vi "Mixed Mode Parameters Dialog.vi"(8 "error in (no error)":errorcluster, 11 "LBCB":T2) -> (0 "error out":errorcluster)   [LabVIEW 2009]
uses:
  lib/Data Access Objects/Metadata/Cartesian Point.ctl
  lib/Data Access Objects/Metadata/Cartesian Force Vector.ctl
  lib/Data Access Objects/Metadata/LBCB Number.ctl
  Update Actions.ctl
  lib/Data Access Objects/Application/Number Of LBCBs.ctl
  lib/Data Access Objects/Metadata/Persistant DAO Actions.ctl
panel:
  out "L2 Default Jacobian Gain":T1
  out "L2 Default Max Increment":T1
  out "L2 Default Force Error Range":T1
  out "L1 Default Jacobian Gain":T1
  out "L1 Default Max Increment":T1
  out "L1 Default Force Error Range":T1
  in  "Cancel":bool
  in  "Ok":bool
  in  "Jacobian\nGain":T3
  in  "Force\nError\nTolerance":T3
  in  "Maximum \nDisplacement\nIncrement":T1
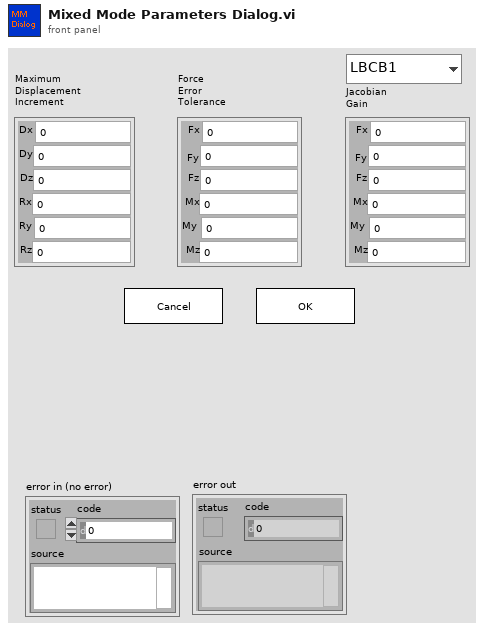
[diagram p1: front panel]
types:
  T1 = typedef "Cartesian Point.ctl" = cluster{"Dx":dbl, "Dy":dbl, "Dz":dbl, "Rx":dbl, "Ry":dbl, "Rz":dbl}
  T2 = typedef "LBCB Number.ctl" = enum16{"LBCB1", "LBCB2"}
  T3 = typedef "Cartesian Force Vector.ctl" = cluster{"Fx":dbl, "Fy":dbl, "Fz":dbl, "Mx":dbl, "My":dbl, "Mz":dbl}
  T4 = typedef "Update Actions.ctl" = enum16{"Update", "Exit"}
  T5 = enum8{"Enabled", "Disabled", "Disabled and Grayed Out"}
  T6 = typedef "Number Of LBCBs.ctl" = enum16{"1", "2"}
  T7 = typedef "Persistant DAO Actions.ctl" = enum16{"Init", "Get", "Set", "Load", "Save"}
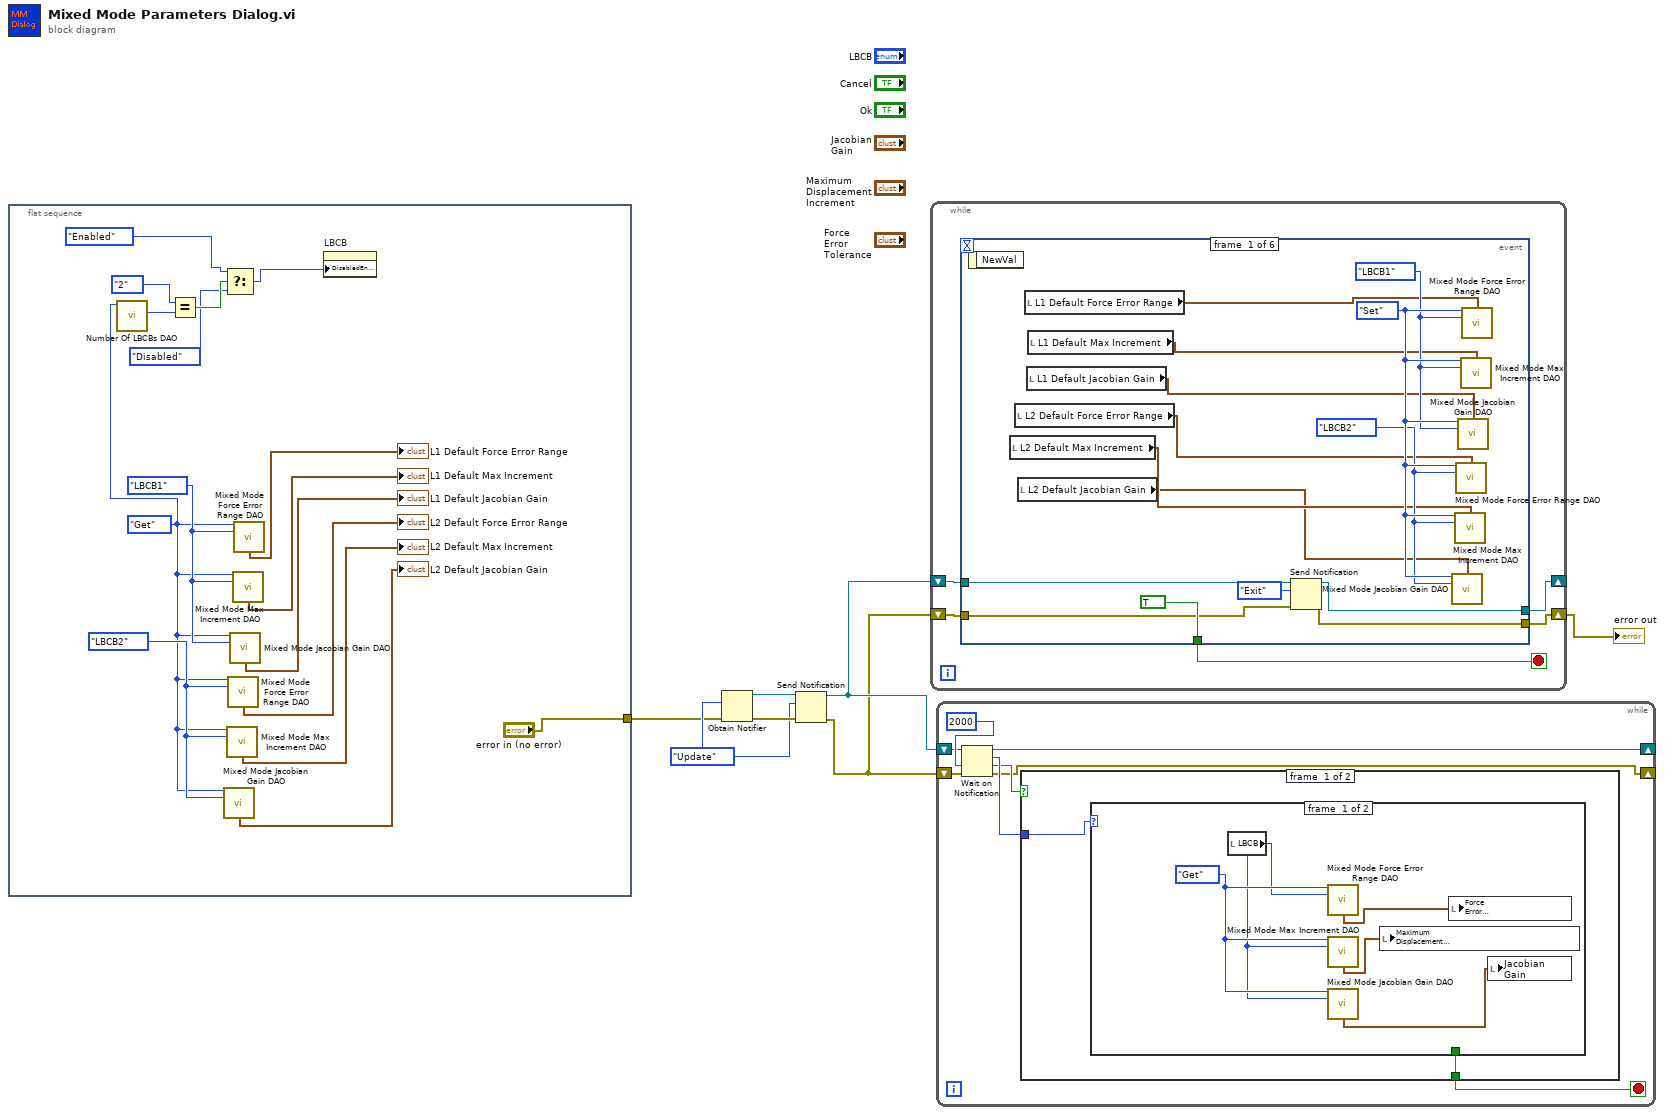
[diagram p0: block diagram]
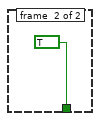
[diagram p2: hidden frame]
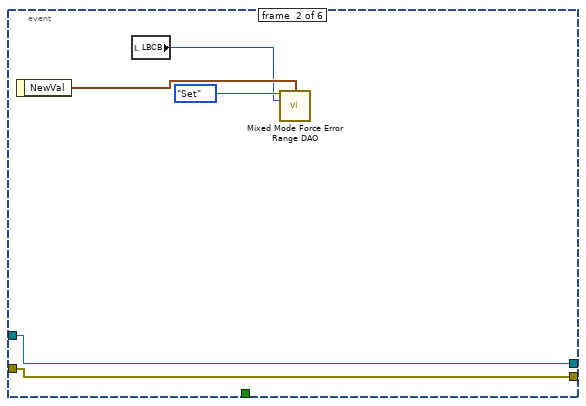
[diagram p4: hidden frame]
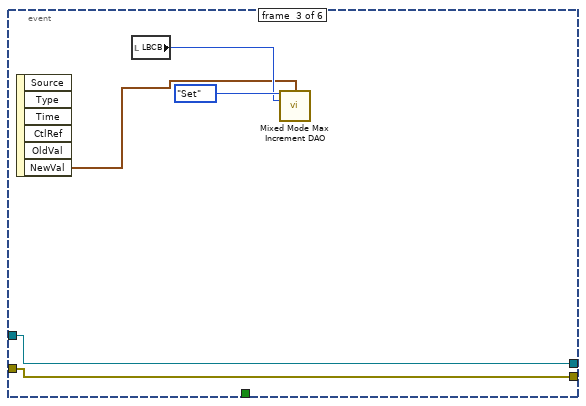
[diagram p5: hidden frame]
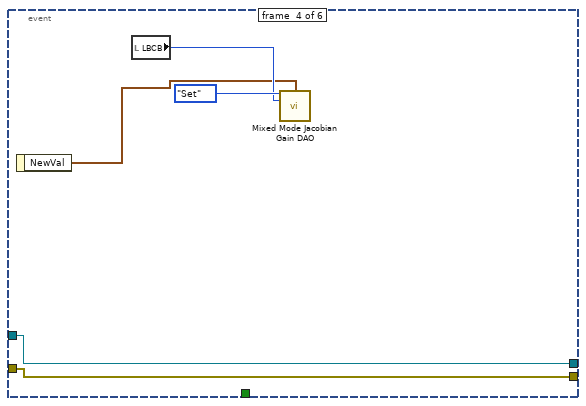
[diagram p6: hidden frame]
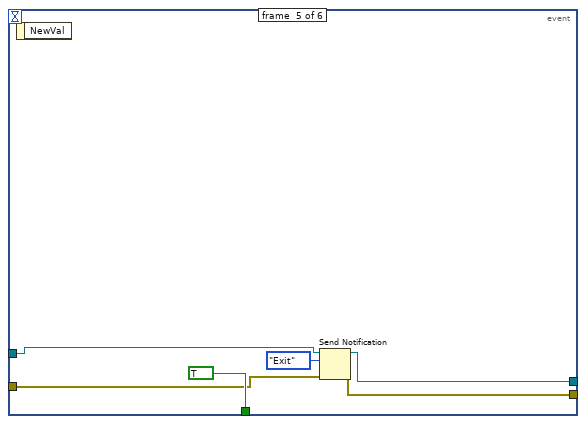
[diagram p7: hidden frame]
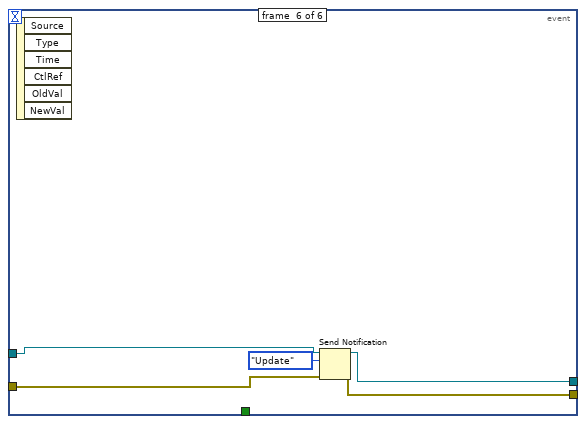
[diagram p8: hidden frame]
diagram:
  w5 = Update_Actions."Update" ("Update Actions")
  n1 = flat-sequence {
    tunnel: ["error in (no error)"] -> w4
    frame #0 {
      w16 = LBCB_Number."LBCB2" ("LBCB Number")
      w20 = LBCB_Number."LBCB1" ("LBCB Number")
      w9 = Persistant_DAO_Actions."Get" ("Force Error Range Actions")
      n2 = call "Number Of LBCBs DAO.vi"("Actions"=w9) -> ("Number of\nLBCBs Out"=w14:T6)  [unwired: 7 in, 3 out]
      n3 = Equal?(x=Number_Of_LBCBs."2", y=w14) -> (x = y?=w12:bool)
      n4 = call "Mixed Mode Jacobian Gain DAO.vi"("Jacobian Gain Actions"=w9, "LBCB Number"=w16) -> ("Jacobian Gain Out"=→"L2 Default Jacobian Gain":T1)  [unwired: 3 in, 10 out]
      n5 = Select(t=T5."Enabled" ("Disabled"), s=w12, f=T5."Disabled") -> (s? t:f=w8:T5)
      n6 = call "Mixed Mode Max Increment DAO.vi"("Max Increment Actions"=w9, "LBCB Number"=w16) -> ("Max Increment Out"=→"L2 Default Max Increment":T1)  [unwired: 3 in, 10 out]
      n7 = call "Mixed Mode Force Error Range DAO.vi"("Force Error Range Actions"=w9, "LBCB Number"=w16) -> ("Force Error Range Out"=→"L2 Default Force Error Range":T1)  [unwired: 3 in, 10 out]
      n8 = call "Mixed Mode Jacobian Gain DAO.vi"("Jacobian Gain Actions"=w9, "LBCB Number"=w20) -> ("Jacobian Gain Out"=→"L1 Default Jacobian Gain":T1)  [unwired: 3 in, 10 out]
      n9 = call "Mixed Mode Max Increment DAO.vi"("Max Increment Actions"=w9, "LBCB Number"=w20) -> ("Max Increment Out"=→"L1 Default Max Increment":T1)  [unwired: 3 in, 10 out]
      n10 = call "Mixed Mode Force Error Range DAO.vi"("Force Error Range Actions"=w9, "LBCB Number"=w20) -> ("Force Error Range Out"=→"L1 Default Force Error Range":T1)  [unwired: 3 in, 10 out]
      n11 = property on="LBCB" class="Enum (strict)"("DisabledEnum"=w8) -> ()  [unwired: 2 in, 2 out]
    }
  }
  n12 = Obtain Notifier(notification data type=w5, error in (no error)=w4) -> (notifier out=w6:refnum<notifier>, error out=w7:errorcluster)  [unwired: 1 in, 2 out]
  n13 = Send Notification(notification=w5, notifier=w6, error in (no error)=w7) -> (notifier out=w3:refnum<notifier>, error out=w2:errorcluster)
  n14 = while {
    shift-right: [w25] -> _
    shift-left: w3 -> [w27]
    shift-right: [w24] -> w1
    shift-left: w2 -> [w26]
    stop <- w28 stop-if-true
    n15 = event shown="[5] \"LBCB\": Value Change" {
      selector: _ -> [_ _ _ _ _ _]
      dyn-events: _ -> [_ _ _ _ _ _]
      timeout: _ -> [_ _ _ _ _ _]
      tunnel: [TRUE _ _ _ TRUE _] -> w28
      tunnel: w27 -> [w32 w45 w51 w56 w62 w68]
      tunnel: w26 -> [w31 w44 w50 w55 w61 w67]
      tunnel: [w30 w45 w51 w56 w60 w66] -> w25
      tunnel: [w29 w44 w50 w55 w59 w65] -> w24
      event #0 {
        w41 = LBCB_Number."LBCB2" ("LBCB Number")
        w40 = LBCB_Number."LBCB1" ("LBCB Number")
        w42 = Persistant_DAO_Actions."Set" ("Force Error Range Actions")
        n16 = event-data() -> ()  [unwired: 2 out]
        n17 = local read "L2 Default Max Increment"() -> (w35:T1)
        n18 = local read "L2 Default Force Error Range"() -> (w36:T1)
        n19 = local read "L2 Default Jacobian Gain"() -> (w34:T1)
        n20 = local read "L1 Default Force Error Range"() -> (w39:T1)
        n21 = local read "L1 Default Jacobian Gain"() -> (w37:T1)
        n22 = local read "L1 Default Max Increment"() -> (w38:T1)
        n23 = Send Notification(notification=Update_Actions."Exit", notifier=w32, error in (no error)=w31) -> (notifier out=w30:refnum<notifier>, error out=w29:errorcluster)
        n24 = call "Mixed Mode Jacobian Gain DAO.vi"("Jacobian Gain Actions"=w42, "Jacobian Gain In"=w34, "LBCB Number"=w41) -> ()  [unwired: 2 in, 11 out]
        n25 = call "Mixed Mode Max Increment DAO.vi"("Max Increment Actions"=w42, "Max Increment In"=w35, "LBCB Number"=w41) -> ()  [unwired: 2 in, 11 out]
        n26 = call "Mixed Mode Force Error Range DAO.vi"("Force Error Range Actions"=w42, "Force Error Range In"=w36, "LBCB Number"=w41) -> ()  [unwired: 2 in, 11 out]
        n27 = call "Mixed Mode Jacobian Gain DAO.vi"("Jacobian Gain Actions"=w42, "Jacobian Gain In"=w37, "LBCB Number"=w40) -> ()  [unwired: 2 in, 11 out]
        n28 = call "Mixed Mode Max Increment DAO.vi"("Max Increment Actions"=w42, "Max Increment In"=w38, "LBCB Number"=w40) -> ()  [unwired: 2 in, 11 out]
        n29 = call "Mixed Mode Force Error Range DAO.vi"("Force Error Range Actions"=w42, "Force Error Range In"=w39, "LBCB Number"=w40) -> ()  [unwired: 2 in, 11 out]
      }
      event #1 {
        n30 = event-data() -> ("NewVal"=w47:T3)  [unwired: 1 out]
        n31 = local read "LBCB"() -> (w46:T2)
        n32 = call "Mixed Mode Force Error Range DAO.vi"("Force Error Range Actions"=Persistant_DAO_Actions."Set", "Force Error Range In"=w47, "LBCB Number"=w46) -> ()  [unwired: 2 in, 11 out]
      }
      event #2 {
        n33 = event-data() -> ("NewVal"=w49:T1)  [unwired: 6 out]
        n34 = local read "LBCB"() -> (w52:T2)
        n35 = call "Mixed Mode Max Increment DAO.vi"("Max Increment Actions"=Persistant_DAO_Actions."Set" ("Force Error Range Actions"), "Max Increment In"=w49, "LBCB Number"=w52) -> ()  [unwired: 2 in, 11 out]
      }
      event #3 {
        n36 = event-data() -> ("NewVal"=w54:T3)  [unwired: 1 out]
        n37 = local read "LBCB"() -> (w57:T2)
        n38 = call "Mixed Mode Jacobian Gain DAO.vi"("Jacobian Gain Actions"=Persistant_DAO_Actions."Set" ("Force Error Range Actions"), "Jacobian Gain In"=w54, "LBCB Number"=w57) -> ()  [unwired: 2 in, 11 out]
      }
      event #4 {
        n39 = event-data() -> ()  [unwired: 2 out]
        n40 = Send Notification(notification=Update_Actions."Exit", notifier=w62, error in (no error)=w61) -> (notifier out=w60:refnum<notifier>, error out=w59:errorcluster)
      }
      event #5 {
        n41 = event-data() -> ()  [unwired: 7 out]
        n42 = Send Notification(notification=Update_Actions."Update", notifier=w68, error in (no error)=w67) -> (notifier out=w66:refnum<notifier>, error out=w65:errorcluster)
      }
    }
  }
  "error out" <- w1
  n43 = while {
    shift-right: [w72] -> _
    shift-left: w3 -> [w75]
    shift-right: [w71] -> _
    shift-left: w2 -> [w76]
    stop <- w70 stop-if-true
    n44 = Wait on Notification(notifier=w75, timeout in ms (-1)=2000, error in (no error)=w76) -> (notifier out=w72:refnum<notifier>, notification=w74:T4, timed out?=w73:bool, error out=w71:errorcluster)  [unwired: 1 out]
    n45 = case shown="False" w73 {
      tunnel: w74 -> [w79 _]
      tunnel: [w78 _] -> w70
      frame #0 {
        n46 = case shown="\"Exit\"" w79 {
          tunnel: [_ TRUE] -> w78
          frame #0 {
            w84 = Persistant_DAO_Actions."Get" ("Force Error Range Actions")
            n47 = local read "LBCB"() -> (w80:T2)
            n48 = call "Mixed Mode Force Error Range DAO.vi"("Force Error Range Actions"=w84, "LBCB Number"=w80) -> ("Force Error Range Out"=w83:T1)  [unwired: 3 in, 10 out]
            n49 = call "Mixed Mode Max Increment DAO.vi"("Max Increment Actions"=w84, "LBCB Number"=w80) -> ("Max Increment Out"=w82:T1)  [unwired: 3 in, 10 out]
            n50 = call "Mixed Mode Jacobian Gain DAO.vi"("Jacobian Gain Actions"=w84, "LBCB Number"=w80) -> ("Jacobian Gain Out"=w81:T1)  [unwired: 3 in, 10 out]
            n51 = local write "Maximum \nDisplacement\nIncrement"(w82) -> ()
            n52 = local write "Force\nError\nTolerance"(w83) -> ()
            n53 = local write "Jacobian\nGain"(w81) -> ()
          }
          frame #1 {
          }
        }
      }
      frame #1 {
      }
    }
  }
